vi "ExecuteTubeGcode.vi"() -> ()   [LabVIEW 2019]
panel:
  out "Current Command":string
  in  "program name and path":path=path "C:/Users/co2_ctl/Documents/sam/Cornell-TFPX-Mechanics/Gantry/flower_tube/gcode/tube_path_relative_rotate90.pgm"
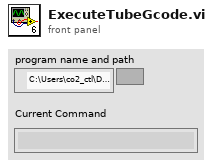
[diagram p1: front panel]
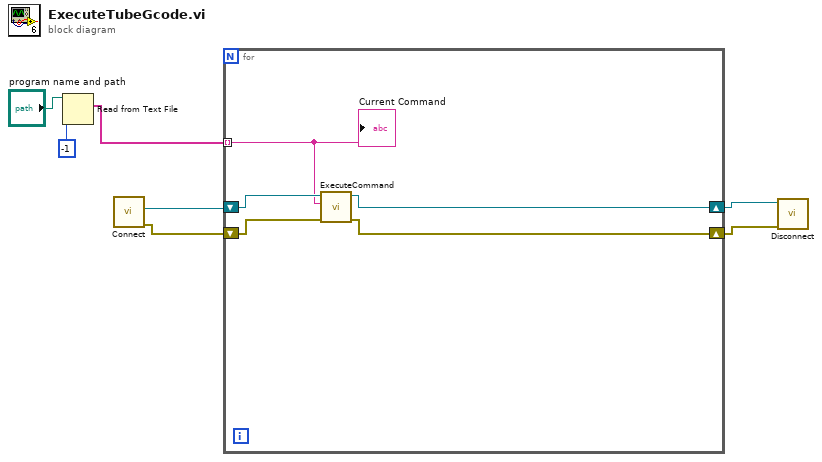
[diagram p0: block diagram]
diagram:
  n1 = Read from Text File(file (use dialog)="program name and path", count=-1) -> (text=w5:string[])  [unwired: 2 in, 3 out]
  n2 = call "Connect.vi"() -> ("error out"=w2:errorcluster, "controller"=w4:refnum<k24>)  [unwired: 10 in]
  n3 = for {
    tunnel: w5 -> [w8] mode=indexing
    shift-right: [w11] -> w3
    shift-left: w4 -> [w12]
    shift-right: [w9] -> w1
    shift-left: w2 -> [w10]
    n4 = call "ExecuteCommand.vi"("error in (no error)"=w10, "Command Code"=w8, "controller in"=w12) -> ("error out"=w9:errorcluster, "controller out"=w11:refnum<k24>)  [unwired: 6 in, 1 out]
    "Current Command" <- w8
  }
  n5 = call "Disconnect.vi"("error in (no error)"=w1, "controller"=w3) -> ()  [unwired: 9 in, 1 out]
